vi "TSPopup.Point to Row Col.vi"(8 "error in (no error)":errorcluster, 9 "Point":cluster{"X":i32, "Y":i32}, 11 "Grid Ctl Reference In":refnum<vi>) -> (0 "error out":errorcluster, 1 "Cell Rect Out":T3={"left"=28, "top"=253, "right"=88, "bottom"=213}, 2 "Cell Info Out":T1, 3 "Grid Ctl Reference Out":refnum<vi>, 4 "In Bounds?":bool)   [LabVIEW 2013]
uses:
  TSPopup.Grid.Cell Info.ctl
  TSPopup.Data Type.ctl
panel:
  in  "Cell Info (type)":T1
  # "Type Sensitive Popup \nCopyright © 2007, J. David Saunders\nAll rights reserved."
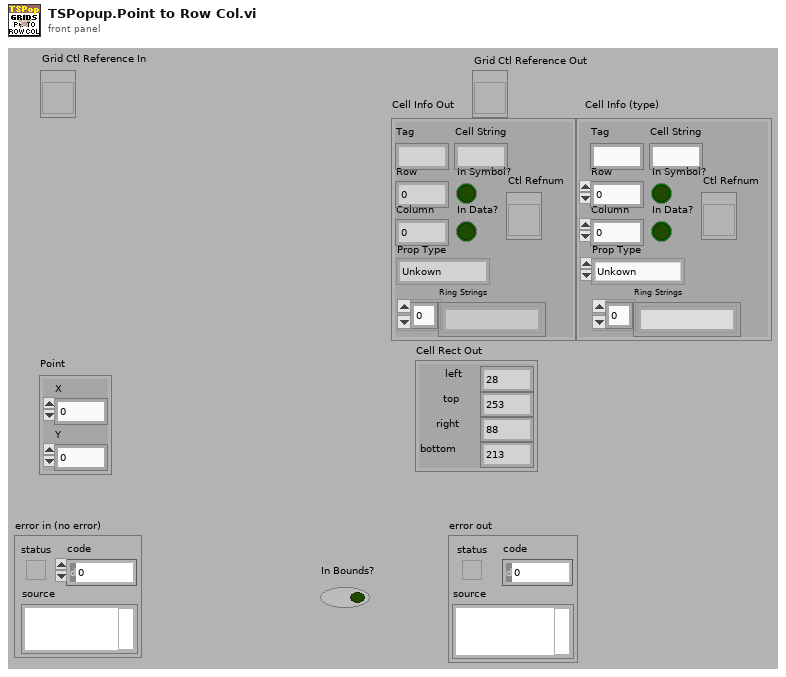
[diagram p1: front panel]
types:
  T1 = typedef "TSPopup.Grid.Cell Info.ctl" = cluster{"Tag":string, "Row":i32, "Column":i32, "In Symbol?":bool, "In Data?":bool, "Cell String":string, "Ctl Refnum":refnum<vi>, "Prop Type":T2, "Ring Strings":string[]}
  T2 = typedef "TSPopup.Data Type.ctl" = enum16{"Unkown", "NO POPUP", "String", "Integer", "Float", "Color", "Boolean", "Ring", "Captioned String", "Captioned Integer", "Button Color", "2 Int Cluster", "4 Int Cluster"}
  T3 = cluster{"left":i16, "top":i16, "right":i16, "bottom":i16}
  T4 = typedef "LVPositionTypeDef.ctl" = cluster{"Left":i32, "Top":i32}
  T5 = typedef "LVRowAndColumnTypeDef.ctl" = cluster{"Row":i32, "Column":i32}
  T6 = typedef "LVBoundsTypeDef.ctl" = cluster{"Width":u32, "Height":u32}
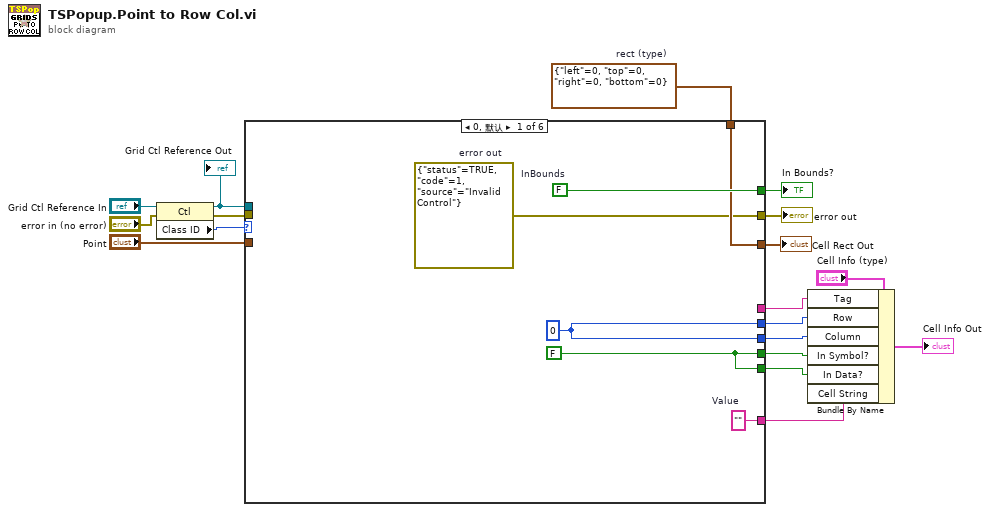
[diagram p0: block diagram]
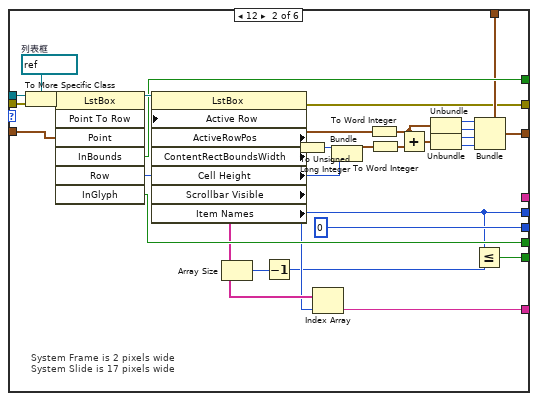
[diagram p2: hidden frame]
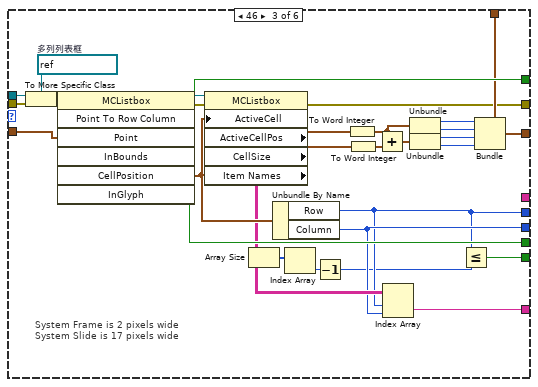
[diagram p3: hidden frame]
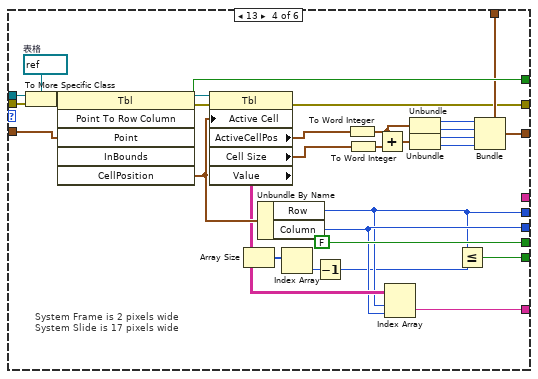
[diagram p4: hidden frame]
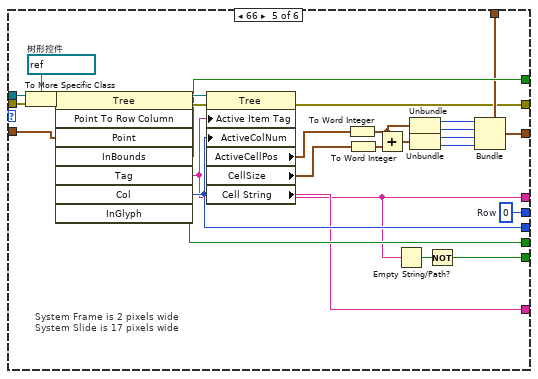
[diagram p5: hidden frame]
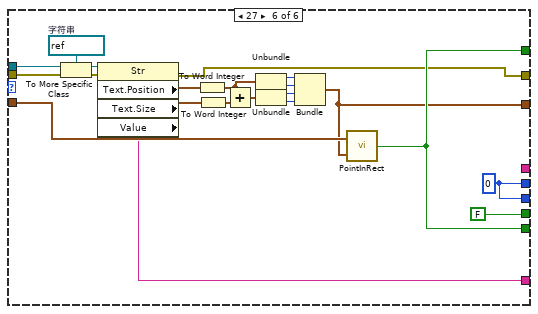
[diagram p6: hidden frame]
diagram:
  w14 = T3 {"left"=0, "top"=0, "right"=0, "bottom"=0}  # rect (type)
  n1 = property class="Ctl"(reference="Grid Ctl Reference In", error in="error in (no error)") -> (reference out=w2:refnum<vi>, error out=w18:errorcluster, "Class ID"=w8:u32)
  "Grid Ctl Reference Out" <- w2
  n2 = case shown="0, 默认" w8 {
    tunnel: w2 -> [_ w53 w84 w115 w143 w151]
    tunnel: w18 -> [_ w52 w83 w114 w142 w150]
    tunnel: [w21 w30 w59 w90 w121 w146] -> w10
    tunnel: "Point" -> [_ w48 w76 w110 w139 w149]
    tunnel: [w23 w29 w58 w89 w124 w165] -> w11
    tunnel: [w23 0 w60 w91 w123 w165] -> w16
    tunnel: [w20 w47 w74 FALSE ("InGlyph") w122 FALSE ("InGlyph")] -> w17
    tunnel: [w22 w33 w64 w93 w125 w145] -> w7
    tunnel: [w24 w46 w75 w107 w136 w148] -> w6
    tunnel: w14 -> [w22 w36 w65 w96 w128 _]
    tunnel: [_ _ _ _ w118 _] -> w12
    tunnel: [w20 w27 w56 w87 w119 w148] -> w9
    tunnel: [w19 w25 w55 w86 w117 w147] -> w3
    frame 0, Default {
      w19 = errorcluster {"status"=TRUE, "code"=1, "source"="Invalid Control"}  # error out
      w21 = ""  # Value
      w20 = FALSE ("InGlyph")
      w24 = FALSE  # InBounds
      w23 = 0
    }
    frame 12 {
      w54 = refnum<vi> refnum  # 列表框
      # "System Frame is 2 pixels wide\nSystem Slide is 17 pixels wide"
      n3 = To More Specific Class(target class=w54, reference=w53, error in=w52) -> (specific class reference=w49:refnum<vi>)  [unwired: 1 out]
      n4 = invoke class="LstBox" method="Point To Row"(reference=w49, "Point"=w48) -> (reference out=w50:refnum<vi>, "InBounds"=w46:bool, "Row"=w29:i32, "InGlyph"=w47:bool)  [unwired: 5 in, 3 out]
      n5 = property on="Property Node" class="LstBox" props=["Active Row", "ActiveRowPos", "ContentRectBoundsWidth", "Cell Height", "Scrollbar Visible", "Item Names"](reference=w50, "Active Row"=w29) -> (error out=w25:errorcluster, "ActiveRowPos"=w35:T4, "ContentRectBoundsWidth"=w45:i32, "Cell Height"=w44:i32, "Item Names"=w31:string[])  [unwired: 1 in, 2 out]
      n6 = Array Size(array=w31) -> (size(s)=w51:i32)
      n7 = Decrement(x=w51) -> (x-1=w28:i32)
      n8 = To Unsigned Long Integer(number=w45) -> (unsigned 32bit integer=w43:u32)
      n9 = Index Array(array=w31, index=w29) -> (element=w30:string)
      n10 = Bundle(w43, "Cell Height"=w44) -> (w34:cluster{u32, "Cell Height":i32})  [unwired: 1 in]
      n11 = To Word Integer(number=w35) -> (16bit integer=w42:cluster{"Left":i16, "Top":i16})
      n12 = To Word Integer(number=w34) -> (16bit integer=w41:cluster{i16, "Cell Height":i16})
      n13 = Add(x=w42, y=w41) -> (x+y=w37:cluster{i16, i16})
      n14 = Unbundle(w42) -> ("Left"=w38:i16, "Top"=w39:i16)
      n15 = Unbundle(w37) -> (w26:i16, w40:i16)
      n16 = Less Or Equal?(x=w29, y=w28) -> (x <= y?=w27:bool)
      n17 = Bundle(cluster=w36, "left"=w38, "top"=w39, "right"=w26, "bottom"=w40) -> (w33:T3)
    }
    frame 46 {
      w85 = refnum<vi> refnum  # 多列列表框
      # "System Frame is 2 pixels wide\nSystem Slide is 17 pixels wide"
      n18 = To More Specific Class(target class=w85, reference=w84, error in=w83) -> (specific class reference=w80:refnum<vi>, error out=w79:errorcluster)
      n19 = invoke class="MCListbox" method="Point To Row Column"(reference=w80, error in=w79, "Point"=w76) -> (reference out=w78:refnum<vi>, error out=w77:errorcluster, "InBounds"=w75:bool, "CellPosition"=w73:T5, "InGlyph"=w74:bool)  [unwired: 4 in, 2 out]
      n20 = property on="Property Node" class="MCListbox"(reference=w78, error in=w77, "ActiveCell"=w73) -> (error out=w55:errorcluster, "ActiveCellPos"=w63:T4, "CellSize"=w62:T6, "Item Names"=w61:string[][])  [unwired: 1 out]
      n21 = Array Size(array=w61) -> (size(s)=w82:i32[])
      n22 = Unbundle By Name(w73) -> ("Row"=w58:i32, "Column"=w60:i32)
      n23 = Index Array(array=w82) -> (element=w81:i32)  [unwired: 1 in]
      n24 = Decrement(x=w81) -> (x-1=w57:i32)
      n25 = To Word Integer(number=w63) -> (16bit integer=w72:cluster{"Left":i16, "Top":i16})
      n26 = To Word Integer(number=w62) -> (16bit integer=w71:cluster{"Width":i16, "Height":i16})
      n27 = Add(x=w72, y=w71) -> (x+y=w66:cluster{i16, i16})
      n28 = Index Array(array=w61, index (row)=w58, index (col)=w60) -> (element=w59:string)
      n29 = Unbundle(w72) -> ("Left"=w67:i16, "Top"=w68:i16)
      n30 = Unbundle(w66) -> (w69:i16, w70:i16)
      n31 = Less Or Equal?(x=w58, y=w57) -> (x <= y?=w56:bool)
      n32 = Bundle(cluster=w65, "left"=w67, "top"=w68, "right"=w69, "bottom"=w70) -> (w64:T3)
    }
    frame 13 {
      w116 = refnum<vi> refnum  # 表格
      # "System Frame is 2 pixels wide\nSystem Slide is 17 pixels wide"
      n33 = To More Specific Class(target class=w116, reference=w115, error in=w114) -> (specific class reference=w112:refnum<vi>, error out=w111:errorcluster)
      n34 = invoke class="Tbl" method="Point To Row Column"(reference=w112, error in=w111, "Point"=w110) -> (reference out=w109:refnum<vi>, error out=w108:errorcluster, "InBounds"=w107:bool, "CellPosition"=w104:T5)  [unwired: 3 in, 2 out]
      n35 = property on="Property Node" class="Tbl"(reference=w109, error in=w108, "Active Cell"=w104) -> (error out=w86:errorcluster, "ActiveCellPos"=w95:T4, "Cell Size"=w94:T6, "Value"=w92:string[][])  [unwired: 1 out]
      n36 = Array Size(array=w92) -> (size(s)=w113:i32[])
      n37 = Unbundle By Name(w104) -> ("Row"=w89:i32, "Column"=w91:i32)
      n38 = Index Array(array=w113) -> (element=w106:i32)  [unwired: 1 in]
      n39 = Decrement(x=w106) -> (x-1=w88:i32)
      n40 = To Word Integer(number=w95) -> (16bit integer=w103:cluster{"Left":i16, "Top":i16})
      n41 = To Word Integer(number=w94) -> (16bit integer=w102:cluster{"Width":i16, "Height":i16})
      n42 = Add(x=w103, y=w102) -> (x+y=w97:cluster{i16, i16})
      n43 = Index Array(array=w92, index (row)=w89, index (col)=w91) -> (element=w90:string)
      n44 = Unbundle(w103) -> ("Left"=w98:i16, "Top"=w99:i16)
      n45 = Unbundle(w97) -> (w100:i16, w101:i16)
      n46 = Less Or Equal?(x=w89, y=w88) -> (x <= y?=w87:bool)
      n47 = Bundle(cluster=w96, "left"=w98, "top"=w99, "right"=w100, "bottom"=w101) -> (w93:T3)
    }
    frame 66 {
      w124 = 0  # Row
      w144 = refnum<vi> refnum  # 树形控件
      # "System Frame is 2 pixels wide\nSystem Slide is 17 pixels wide"
      n48 = To More Specific Class(target class=w144, reference=w143, error in=w142) -> (specific class reference=w141:refnum<vi>, error out=w140:errorcluster)
      n49 = invoke class="Tree" method="Point To Row Column"(reference=w141, error in=w140, "Point"=w139) -> (reference out=w138:refnum<vi>, error out=w137:errorcluster, "InBounds"=w136:bool, "Tag"=w118:string, "Col"=w123:i32, "InGlyph"=w122:bool)  [unwired: 5 in, 2 out]
      n50 = property on="Property Node" class="Tree"(reference=w138, error in=w137, "Active Item Tag"=w118, "ActiveColNum"=w123) -> (error out=w117:errorcluster, "ActiveCellPos"=w127:T4, "CellSize"=w126:T6, "Cell String"=w121:string)  [unwired: 1 out]
      n51 = To Word Integer(number=w127) -> (16bit integer=w135:cluster{"Left":i16, "Top":i16})
      n52 = To Word Integer(number=w126) -> (16bit integer=w134:cluster{"Width":i16, "Height":i16})
      n53 = Add(x=w135, y=w134) -> (x+y=w129:cluster{i16, i16})
      n54 = Empty String/Path?(string/path=w118) -> (empty?=w120:bool)
      n55 = Unbundle(w135) -> ("Left"=w130:i16, "Top"=w131:i16)
      n56 = Unbundle(w129) -> (w132:i16, w133:i16)
      n57 = Not(x=w120) -> (.not. x?=w119:bool)
      n58 = Bundle(cluster=w128, "left"=w130, "top"=w131, "right"=w132, "bottom"=w133) -> (w125:T3)
    }
    frame 27 {
      w152 = refnum<vi> refnum  # 字符串
      w165 = 0 ("Row")
      n59 = To More Specific Class(target class=w152, reference=w151, error in=w150) -> (specific class reference=w153:refnum<vi>, error out=w154:errorcluster)
      n60 = property class="Str"(reference=w153, error in=w154) -> (error out=w147:errorcluster, "Text.Position"=w155:T4, "Text.Size"=w156:T6, "Value"=w146:string)  [unwired: 1 out]
      n61 = To Word Integer(number=w155) -> (16bit integer=w163:cluster{"Left":i16, "Top":i16})
      n62 = To Word Integer(number=w156) -> (16bit integer=w157:cluster{"Width":i16, "Height":i16})
      n63 = Add(x=w163, y=w157) -> (x+y=w162:cluster{i16, i16})
      n64 = Unbundle(w163) -> ("Left"=w161:i16, "Top"=w160:i16)
      n65 = Unbundle(w162) -> (w159:i16, w158:i16)
      n66 = Bundle("Left"=w161, "Top"=w160, w159, w158) -> (w145:cluster{"Left":i16, "Top":i16, i16, i16})  [unwired: 1 in]
      n67 = call <vilib>:"PointInRect.vi"("rect"=w145, "point"=w149) -> ("pt in rect"=w148:bool)
    }
  }
  "In Bounds?" <- w6
  "error out" <- w3
  "Cell Rect Out" <- w7
  n68 = Bundle By Name(cluster="Cell Info (type)", "Tag"=w12, "Row"=w11, "Column"=w16, "In Symbol?"=w17, "In Data?"=w9, "Cell String"=w10) -> (→"Cell Info Out":T1)
